vi "MultiCha-TransmitReceive.vi"() -> ()   [LabVIEW 2023]
uses:
  <instrlib>/BTICardLib/Private/Initialize By Card Number and Core Number.vi
  <instrlib>/BTICardLib/Private/Configure Core From XML.vi
  <instrlib>/BTI429Lib/Private/Tx/Configure/Configure Tx Channel From XML.vi
  <instrlib>/BTI429Lib/Private/Rx/Configure/Configure Rx Channel From XML.vi
  <instrlib>/BTI429Lib/Private/Core/Action-Status/Start All Channels.vi
  <instrlib>/BTI429Lib/Private/Core/Action-Status/Stop All Channels.vi
  <instrlib>/BTI429Lib/Private/Rx/Configure/Get Rx Label Handle Name.vi
  <instrlib>/BTI429Lib/Private/Utility/Get BNR Mantissa.vi
  <instrlib>/BTICardLib/BTICardLV.lvlib
  <instrlib>/BTI429Lib/BTI429LV.lvlib
panel:
  out "Label3Value":u32 format="%08x"
  out "Label2Value":u32 format="%08x"
  out "mantissa out":u32 format="%08x"
  out "Label1Value":u32 format="%08x"
  in  "stop":bool
  out "error out":errorcluster
  in  "Rx channel number":i32=3
  out "Channel Rx Xml Path":path
  in  "Channel Configuration Rx XML file name":string="Channel Config.xml"
  in  "Tx channel number":i32=18
  out "Core Xml Path":path
  out "Channel Tx Xml Path":path
  in  "Core Configuration XML file name":string="Core Config.xml"
  in  "Channel ConfigurationTx XML file name":string="Channel Config.xml"
  in  "core number":i32
  in  "card number":i32
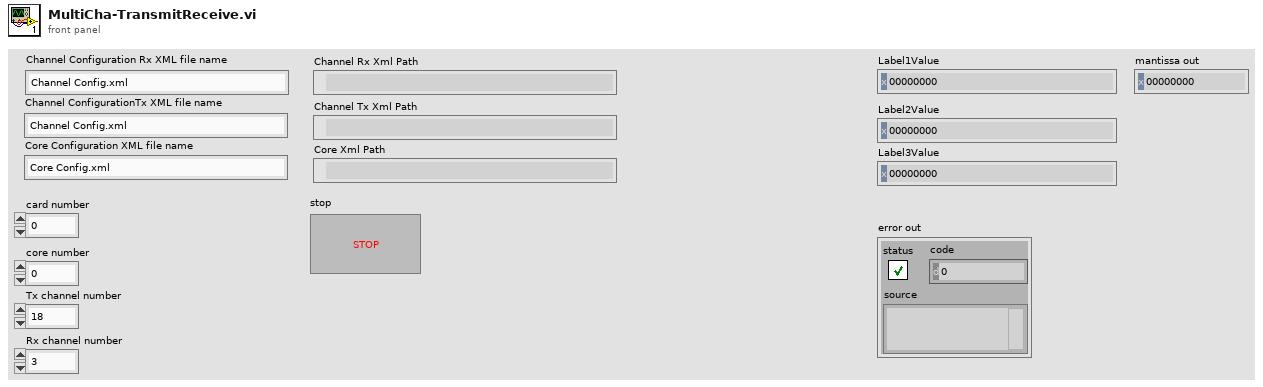
[diagram p1: front panel]
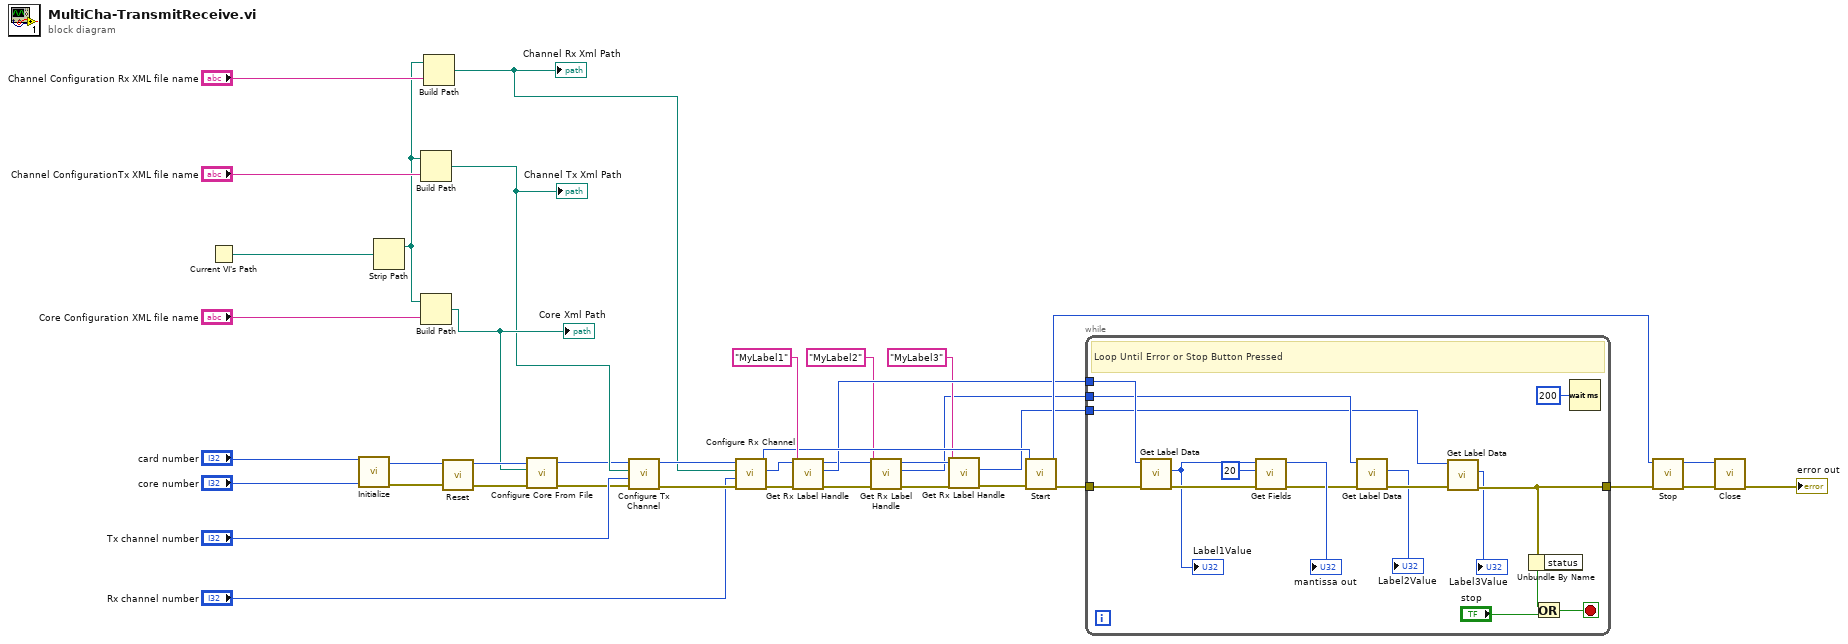
[diagram p0: block diagram]
diagram:
  n1 = Current VI's Path() -> (path=w35:path)
  n2 = call-poly <instrlib>:"Initialize.vi"("core number"="core number", "card number"="card number") -> ("error out"=w37:errorcluster, "core handle out"=w38:u64)  [unwired: 8 in]
  n3 = Strip Path(path=w35) -> (stripped path=w24:path)  [unwired: 1 out]
  n4 = Build Path(base path=w24, name or relative path="Channel ConfigurationTx XML file name") -> (appended path=w31:path)
  "Channel Tx Xml Path" <- w31
  n5 = Build Path(base path=w24, name or relative path="Core Configuration XML file name") -> (appended path=w32:path)
  "Core Xml Path" <- w32
  n6 = Build Path(base path=w24, name or relative path="Channel Configuration Rx XML file name") -> (appended path=w23:path)
  "Channel Rx Xml Path" <- w23
  n7 = call <instrlib>:"Reset.vi"("error in (no error)"=w37, "core handle in"=w38) -> ("error out"=w28:errorcluster, "core handle out"=w36:u64)  [unwired: 8 in]
  n8 = call-poly <instrlib>:"Configure Core From File.vi"("error in (no error)"=w28, "configuration file path"=w32, "core handle in"=w36) -> ("error out"=w27:errorcluster, "core handle out"=w30:u64)  [unwired: 7 in]
  n9 = call-poly <instrlib>:"Configure Tx Channel.vi"("error in (no error)"=w27, "channel number in"="Tx channel number", "configuration file path"=w31, "core handle in"=w30) -> ("error out"=w22:errorcluster, "core handle out"=w26:u64)  [unwired: 5 in, 1 out]
  n10 = call-poly <instrlib>:"Configure Rx Channel.vi"("error in (no error)"=w22, "channel number in"="Rx channel number", "configuration file path"=w23, "core handle in"=w26) -> ("error out"=w19:errorcluster, "channel handle out"=w20:u64, "core handle out"=w13:u64)  [unwired: 5 in]
  n11 = call-poly <instrlib>:"Get Rx Label Handle.vi"("error in (no error)"=w19, "label name"="MyLabel1", "channel handle in"=w20) -> ("error out"=w7:errorcluster, "label handle out"=w12:u64, "channel handle out"=w5:u64)  [unwired: 6 in]
  n12 = call-poly <instrlib>:"Get Rx Label Handle.vi"("error in (no error)"=w7, "label name"="MyLabel2", "channel handle in"=w5) -> ("error out"=w9:errorcluster, "label handle out"=w2:u64, "channel handle out"=w8:u64)  [unwired: 6 in]
  n13 = call-poly <instrlib>:"Get Rx Label Handle.vi"("error in (no error)"=w9, "label name"="MyLabel3", "channel handle in"=w8) -> ("error out"=w6:errorcluster, "label handle out"=w1:u64)  [unwired: 6 in, 1 out]
  n14 = call-poly <instrlib>:"Start.vi"("error in (no error)"=w6, "core handle in"=w13) -> ("error out"=w11:errorcluster, "core handle out"=w17:u64)  [unwired: 8 in]
  n15 = while {
    tunnel: w12 -> [w54]
    tunnel: w11 -> [w55]
    tunnel: [w44] -> w10
    tunnel: w2 -> [w46]
    tunnel: w1 -> [w43]
    stop <- w57 stop-if-true
    # "Loop Until Error or Stop Button Pressed"
    n16 = call <instrlib>:"Get Label Data.vi"("error in (no error)"=w55, "label handle in"=w54) -> ("error out"=w50:errorcluster, "value"=w49:u32)  [unwired: 7 in, 1 out]
    "Label1Value" <- w49
    n17 = call-poly <instrlib>:"Get Fields.vi"("error in (no error)"=w50, "significant digits"=u16 20 ("most significant bit"), "message"=w49) -> ("error out"=w47:errorcluster, "mantissa out"=→"mantissa out":u32)  [unwired: 7 in]
    n18 = call <instrlib>:"Get Label Data.vi"("error in (no error)"=w47, "label handle in"=w46) -> ("error out"=w45:errorcluster, "value"=→"Label2Value":u32)  [unwired: 7 in, 1 out]
    n19 = call <instrlib>:"Get Label Data.vi"("error in (no error)"=w45, "label handle in"=w43) -> ("error out"=w44:errorcluster, "value"=→"Label3Value":u32)  [unwired: 7 in, 1 out]
    n20 = Unbundle By Name(w44) -> ("status"=w53:bool)
    n21 = Or(x=w53, y="stop") -> (x .or. y?=w57:bool)
    n22 = Wait (ms)(milliseconds to wait=u32 200) -> ()  [unwired: 1 out]
  }
  n23 = call-poly <instrlib>:"Stop.vi"("error in (no error)"=w10, "core handle in"=w17) -> ("error out"=w15:errorcluster, "core handle out"=w16:u64)  [unwired: 8 in]
  n24 = call <instrlib>:"Close.vi"("error in (no error)"=w15, "core handle in"=w16) -> ("error out"=→"error out":errorcluster)  [unwired: 8 in, 1 out]
